vi "PC_DCG to DFM.vi"() -> ()   [LabVIEW 2021]
uses:
  Digital Frequency Measurement/Typedefs/Range Settings.ctl
  Digital Clock Generation/Typedefs/Digital Clock Settings.ctl
  Digital Clock Generation/Typedefs/Actual Clock Settings.ctl
  Digital Frequency Measurement/DAQ_Digital Frequency Measurement.lvlib
  Digital Clock Generation/DAQ_Digital Clock Generation.lvlib
panel:
  out "error out":errorcluster
  out "Detected Frequency (Hz)":dbl=99999.99999999999 format="%.6p"
  out "Actual Clock Settings":T1={"Frequency (Hz)"=100000.0, "Duty Cycle (%)"=50.0, "Generation Time (s)"=0.1} {"Duty Cycle (%)" format="%#.2p"; "Frequency (Hz)" format="%.6p"; "Generation Time (s)" format="%.2p"}
  in  "Digital Clock Settings":T2={"Frequency (Hz)"=100000.0, "Duty Cycle(%)"=50.0, "Generation Time (s)"=0.1} {"Duty Cycle(%)" format="%#.2p"; "Frequency (Hz)" format="%.6p"; "Generation Time (s)" format="%.2p"}
  in  "Input Frequency Divisor":u32=4 min=4 step=1
  in  "Range Settings":T3={"Max Frequency (Hz)"=20000000.0, "Min Frequency (Hz)"=1.0} {"Min Frequency (Hz)" format="%.6p"; "Max Frequency (Hz)" format="%.6p"}
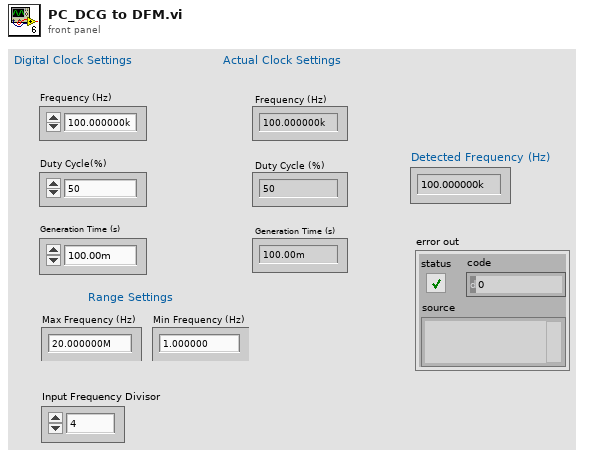
[diagram p1: front panel]
types:
  T1 = typedef "DAQ_Digital Clock Generation.lvlib/Actual Clock Settings.ctl" = cluster{"Frequency (Hz)":dbl, "Duty Cycle (%)":dbl, "Generation Time (s)":dbl}
  T2 = typedef "DAQ_Digital Clock Generation.lvlib/Digital Clock Settings.ctl" = cluster{"Frequency (Hz)":dbl, "Duty Cycle(%)":dbl, "Generation Time (s)":dbl}
  T3 = typedef "DAQ_Digital Frequency Measurement.lvlib/Range Settings.ctl" = cluster{"Max Frequency (Hz)":dbl, "Min Frequency (Hz)":dbl}
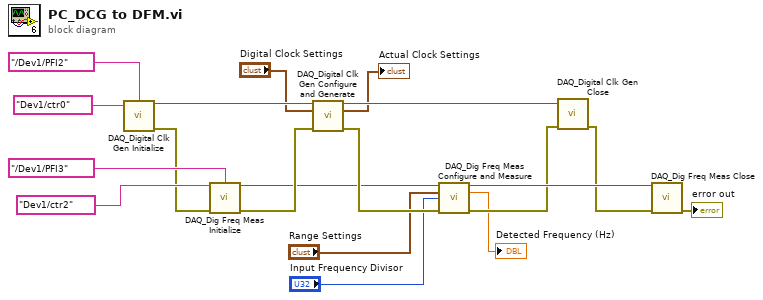
[diagram p0: block diagram]
diagram:
  n1 = call "DAQ_Digital Clk Gen Initialize.vi"("Physical Channel (Counter)"=tag "Dev1/ctr0", "Output Terminal"=tag "/Dev1/PFI2") -> ("DAQmx Task Out"=w12:refnum<k21>, "error out"=w15:errorcluster)  [unwired: 12 in]
  n2 = call "DAQ_Dig Freq Meas Initialize.vi"("Physical Channel (counter)"=tag "Dev1/ctr2", "Input Terminal"=tag "/Dev1/PFI3", "error in"=w15) -> ("DAQmx Task Out"=w10:refnum<k21>, "error out"=w14:errorcluster)  [unwired: 11 in]
  n3 = call "DAQ_Digital Clk Gen Configure and Generate.vi"("DAQmx Task In"=w12, "Digital Clock Settings"="Digital Clock Settings", "error in"=w14) -> ("DAQmx Task Out"=w11:refnum<k21>, "Actual Clock Settings"=→"Actual Clock Settings":T1, "error out"=w13:errorcluster)  [unwired: 10 in]
  n4 = call "DAQ_Dig Freq Meas Configure and Measure.vi"("DAQmx Task In"=w10, "Range Settings"="Range Settings", "Input Frequency Divisor"="Input Frequency Divisor", "error in"=w13) -> ("DAQmx Task Out"=w9:refnum<k21>, "Detected Frequency (Hz)"=→"Detected Frequency (Hz)":dbl, "error out"=w8:errorcluster)  [unwired: 9 in]
  n5 = call "DAQ_Digital Clk Gen Close.vi"("DAQmx Task In"=w11, "error in"=w8) -> ("error out"=w7:errorcluster)  [unwired: 13 in]
  n6 = call "DAQ_Dig Freq Meas Close.vi"("DAQmx Task In"=w9, "error in"=w7) -> ("error out"=→"error out":errorcluster)  [unwired: 13 in]
